vi "Array2tdmStr.vi"(11 "Array":dbl[](array[numeric])) -> (3 "String":string)   [LabVIEW 2023]
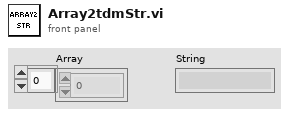
[diagram p1: front panel]
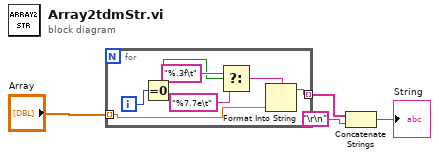
[diagram p0: block diagram]
diagram:
  n1 = for {
    tunnel: [w11] -> w1 mode=indexing
    tunnel: "Array" -> [w5] mode=indexing
    i -> [w7]
    n2 = Equal To 0?(x=w7) -> (x = 0?=w6:bool)
    n3 = Select(t="%.3f\t" ("format string"), s=w6, f="%7.7e\t" ("format string")) -> (s? t:f=w8:string)
    n4 = Format Into String(format string=w8, w5) -> (resulting string=w11:string)  [unwired: 2 in, 1 out]
  }
  n5 = Concatenate Strings(w1, "\r\n") -> (→"String":string)
